vi "Tosca-Process Autoscale Change.vi"(0 "state in":T1, 7 "autoscale":bool) -> (4 "state out":T1)   [LabVIEW 2020]
uses:
  Typedefs/Tosca-AI UI State.ctl
  Typedefs/Tosca-AI Plot Properties.ctl
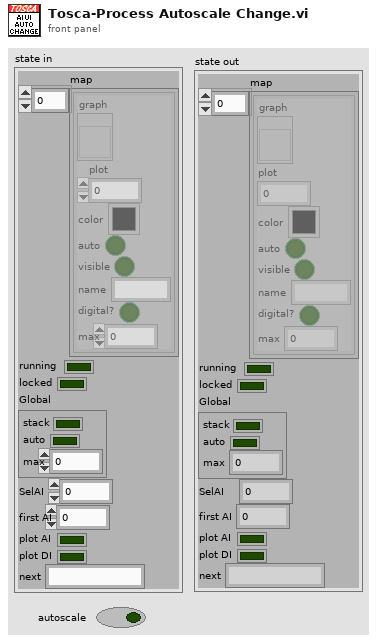
[diagram p1: front panel]
types:
  T1 = typedef "Tosca-AI UI State.ctl" = cluster{"map":T2[], "running":bool, "locked":bool, "Global":cluster{"stack":bool, "auto":bool, "max":dbl}, "SelAI":i32, "first AI":i32, "plot AI":bool, "plot DI":bool, "next":string}
  T2 = typedef "Tosca-AI Plot Properties.ctl" = cluster{"graph":refnum<vi>, "plot":i32, "color":u32, "auto":bool, "visible":bool, "name":string, "digital?":bool, "max":dbl}
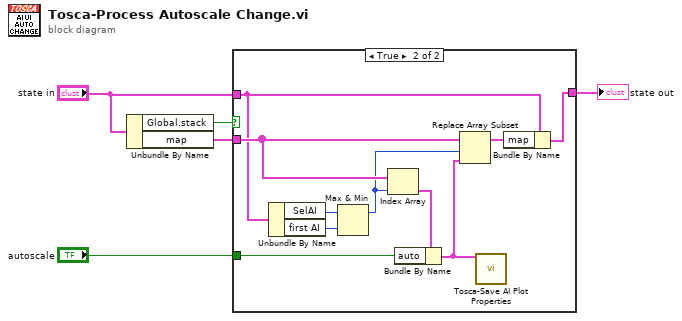
[diagram p0: block diagram]
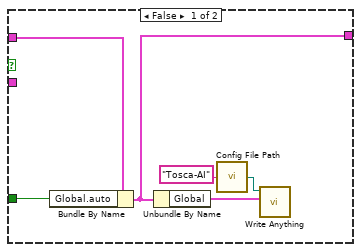
[diagram p2: hidden frame]
diagram:
  n1 = Unbundle By Name("state in") -> ("Global.stack"=w2:bool, "map"=w5:T2[])
  n2 = case shown="True" w2 {
    tunnel: w5 -> [_ w20]
    tunnel: "state in" -> [w11 w16]
    tunnel: [w6 w19] -> w3
    tunnel: "autoscale" -> [w10 w13]
    frame False {
      n3 = Bundle By Name(cluster=w11, "Global.auto"=w10) -> (w6:T1)
      n4 = Unbundle By Name(w6) -> ("Global"=w7:cluster{"stack":bool, "auto":bool, "max":dbl})
      n5 = call "Config File Path.vi"("AppName"="Tosca-AI") -> ("Default config file name"=w9:path)
      n6 = call "Write Anything.vi"("Anything"=w7, "Path (dialog)"=w9) -> ()  [unwired: 8 in, 2 out]
    }
    frame True {
      n7 = Unbundle By Name(w16) -> ("SelAI"=w15:i32, "first AI"=w14:i32)
      n8 = Max & Min(x=w15, y=w14) -> (max(x,y)=w12:i32)  [unwired: 1 out]
      n9 = Index Array(array=w20, index=w12) -> (element=w21:T2)
      n10 = Bundle By Name(cluster=w21, "auto"=w13) -> (w17:T2)
      n11 = Replace Array Subset(array=w20, new element=w17, index=w12) -> (w18:T2[])
      n12 = call "Tosca-Save AI Plot Properties.vi"("plot"=w17) -> ()  [unwired: 15 in]
      n13 = Bundle By Name(cluster=w16, "map"=w18) -> (w19:T1)
    }
  }
  "state out" <- w3
